vi "test_RxUDP.vi"() -> ()   [LabVIEW 2020]
uses:
  <instrlib>/AIM GmbH/_AIM 664/_controls/comm_computedMAC-IP.ctl
  <instrlib>/AIM GmbH/_AIM 664/_controls/comm_verification_rx.ctl
  <instrlib>/AIM GmbH/_AIM 664/_controls/comm_udp_rx.ctl
  <instrlib>/AIM GmbH/_AIM 664/bsp/Controls/IrigTime.ctl
  <instrlib>/AIM GmbH/_AIM 664/bsp/Fdx Create Session (Rx-VL-Oriented).vi
  <instrlib>/AIM GmbH/_AIM 664/bsp/Receive/FdxCreateRxVL.vi
  <instrlib>/AIM GmbH/_AIM 664/bsp/Fdx Create UDP Port (RX-CommPort).vi
  <instrlib>/AIM GmbH/_AIM 664/bsp/Fdx Start (Rx).vi
  <instrlib>/AIM GmbH/_AIM 664/bsp/TargetIndependentAdmin/FdxFwIrig2StructIrig.vi
  <instrlib>/AIM GmbH/_AIM 664/bsp/Fdx Stop (Rx).vi
  <instrlib>/AIM GmbH/_AIM 664/AIM664LV.lvlib
panel:
  out "IrigTime out":T1
  out "Udp Message":u8[](array[numeric]) format="%.0x"
  out "time stamp":timestamp
  out "timestamp s":dbl format="%#_15g"
  out "read time uS":u32(graph)
  out "MsgRead Total":u32=2
  in  "rx fetch rate mS":u32=100
  out "GlobalStat Out":T2={"TotalByteCount"=[139198, 0, 0, 0, 0, 0, 0, 0], "FrameGoodCount"=[1762, 0, 0, 0, 0, 0, 0, 0], "FrameErrorCount"=[0, 0, 0, 0, 0, 0, 0, 0], "BytesPerSecond"=[15800, 0, 0, 0, 0, 0, 0, 0], "FramesPerSecond"=[200, 0, 0, 0, 0, 0, 0, 0], "PhysErrorCount"=[0, 0, 0, 0, 0, 0, 0, 0], "PreamErrorCount"=[0, 0, 0, 0, 0, 0, 0, 0], "UnaligErrorCount"=[0, 0, 0, 0, 0, 0, 0, 0], "CRCErrorCount"=[0, 0, 0, 0, 0, 0, 0, 0], "IFGErrorCount"=[0, 0, 0, 0, 0, 0, 0, 0], "IPErrorCount"=[0, 0, 0, 0, 0, 0, 0, 0], "MACErrorCount"=[0, 0, 0, 0, 0, 0, 0, 0], "NoSfdErrorCount"=[0, 0, 0, 0, 0, 0, 0, 0], "VLLenErrorCount"=[0, 0, 0, 0, 0, 0, 0, 0], "SNIntegrityErrorCount"=[0, 0, 0, 0, 0, 0, 0, 0], "TrafShapingViolationCount"=[0, 0, 0, 0, 0, 0, 0, 0], "MAC1Short"=[0, 0, 0, 0, 0, 0, 0, 0], "MAC64To127Count"=[1762, 0, 0, 0, 0, 0, 0, 0], "MAC128To255Count"=[0, 0, 0, 0, 0, 0, 0, 0], "MAC256To511Count"=[0, 0, 0, 0, 0, 0, 0, 0], "MAC512To1023Count"=[0, 0, 0, 0, 0, 0, 0, 0], "MAC1024To1518Count"=[0, 0, 0, 0, 0, 0, 0, 0], "MACLong"=[0, 0, 0, 0, 0, 0, 0, 0]}
  in  "Control":u32(ring) items=["FDX_RX_GS_RES_NO_CNT", "FDX_RX_GS_RES_ALL_CNT", "FDX_RX_GS_RES_ERR_CNT"]
  out "MsgRead":u32=2
  out "MsgCount":u32=1762
  out "MsgErrorCount":u32
  out "RxStatus":u32=1
  out "Info":u32
  in  "stop":bool
  in  "Array":T3[](array[typedef])=[{"PortType"=enum."FDX_UDP_SAMPLING", "SubVIId"=1, "domainID"=1, "sideID"=1, "locationID"=1, "partitionID"=1, "UdpSrcPort"=24, "UdpDstPort"=23, "UdpNumBufMessages"=1, "UdpMaxMessageSize"=512, "UdpSamplingRate"=0}] {"partitionID" format="%.0b"}
  in  "VL Config":T4={"VlId"=60, "VLRange"=1, "VerificationMode"=0, "Bag"=0, "Jitter"=0, "MaxFrameLength"=0, "MaxSkew"=0, "VLBufSize"=32768, "FilterMode"=0, "FilterPosition"=0, "Padding"=0, "FilterMask"=0, "FilterData"=0, "MinFrameLength"=0} {"FilterMode" items=["FDX_RX_VL_FLT_DIS", "FDX_RX_VL_FLT_ENA ", "FDX_RX_VL_FLT_ENA_INV"]; "VLBufSize" format="%.0x"; "MaxFrameLength" format="%.0x"; "VerificationMode" items=["FDX_RX_VL_CHECK_ENA_DEFAULT"=65535, "FDX_RX_VL_CHECK_REDMAM"=16, "DX_RX_VL_CHECK_TRAFIC"=8, "FDX_RX_VL_CHECK_FRAMESIZE"=4, "FDX_RX_VL_CHECK_SNINTEG"=2, "FDX_RX_VL_CHECK_INVPAC"=1, "FDX_RX_VL_CHECK_DISA"=0]}
  out "computedAddresses":T5={"MACsrc"=[2, 0, 0, 1, 33, 32], "IPsrc"="10.1.33.1", "IPdest"="224.224.0.60"} {"MACsrc" format="%.0x"}
  in  "PortMap":u32=2
  out "PortInitOut":T6={"PortConfig"=0, "PortUsed"=1, "GlobalMemFree"=0, "SharedMemFree"=0} {"PortConfig" items=["FDX_SINGLE", "FDX_REDUNDANT"]}
  in  "port":u32
  in  "board":u32=1
  out "error out":errorcluster
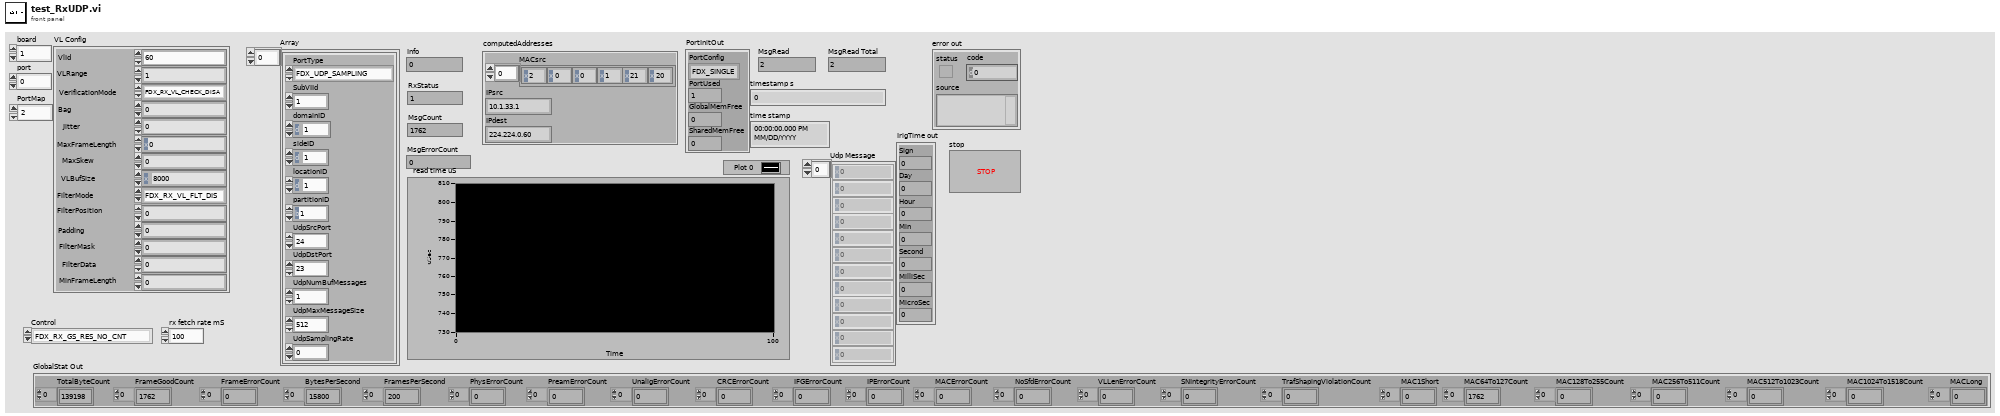
[diagram p1: front panel]
types:
  T1 = typedef "AIM664LV.lvlib/IrigTime.ctl" = cluster{"Sign":i32, "Day":u32, "Hour":u32, "Min":u32, "Second":u32, "MilliSec":u32, "MicroSec":u32}
  T2 = cluster{"TotalByteCount":u32[], "FrameGoodCount":u32[], "FrameErrorCount":u32[], "BytesPerSecond":u32[], "FramesPerSecond":u32[], "PhysErrorCount":u32[], "PreamErrorCount":u32[], "UnaligErrorCount":u32[], "CRCErrorCount":u32[], "IFGErrorCount":u32[], "IPErrorCount":u32[], "MACErrorCount":u32[], "NoSfdErrorCount":u32[], "VLLenErrorCount":u32[], "SNIntegrityErrorCount":u32[], "TrafShapingViolationCount":u32[], "MAC1Short":u32[], "MAC64To127Count":u32[], "MAC128To255Count":u32[], "MAC256To511Count":u32[], "MAC512To1023Count":u32[], "MAC1024To1518Count":u32[], "MACLong":u32[]}
  T3 = typedef "AIM664LV.lvlib/comm_udp_rx.ctl" = cluster{"PortType":enum16{"FDX_UDP_SAMPLING", "FDX_UDP_QUEUING"}, "SubVIId":u32, "domainID":u8, "sideID":u8, "locationID":u8, "partitionID":u8, "UdpSrcPort":u16, "UdpDstPort":u16, "UdpNumBufMessages":u32, "UdpMaxMessageSize":u32, "UdpSamplingRate":u32}
  T4 = typedef "AIM664LV.lvlib/comm_verification_rx.ctl" = cluster{"VlId":u16, "VLRange":u32, "VerificationMode":u32, "Bag":u32, "Jitter":u32, "MaxFrameLength":u32, "MaxSkew":u32, "VLBufSize":u32, "FilterMode":u32, "FilterPosition":u32, "Padding":u32, "FilterMask":u32, "FilterData":u32, "MinFrameLength":u32}
  T5 = typedef "AIM664LV.lvlib/comm_computedMAC-IP.ctl" = cluster{"MACsrc":u8[], "IPsrc":string, "IPdest":string}
  T6 = cluster{"PortConfig":u32, "PortUsed":u32, "GlobalMemFree":u32, "SharedMemFree":u32}
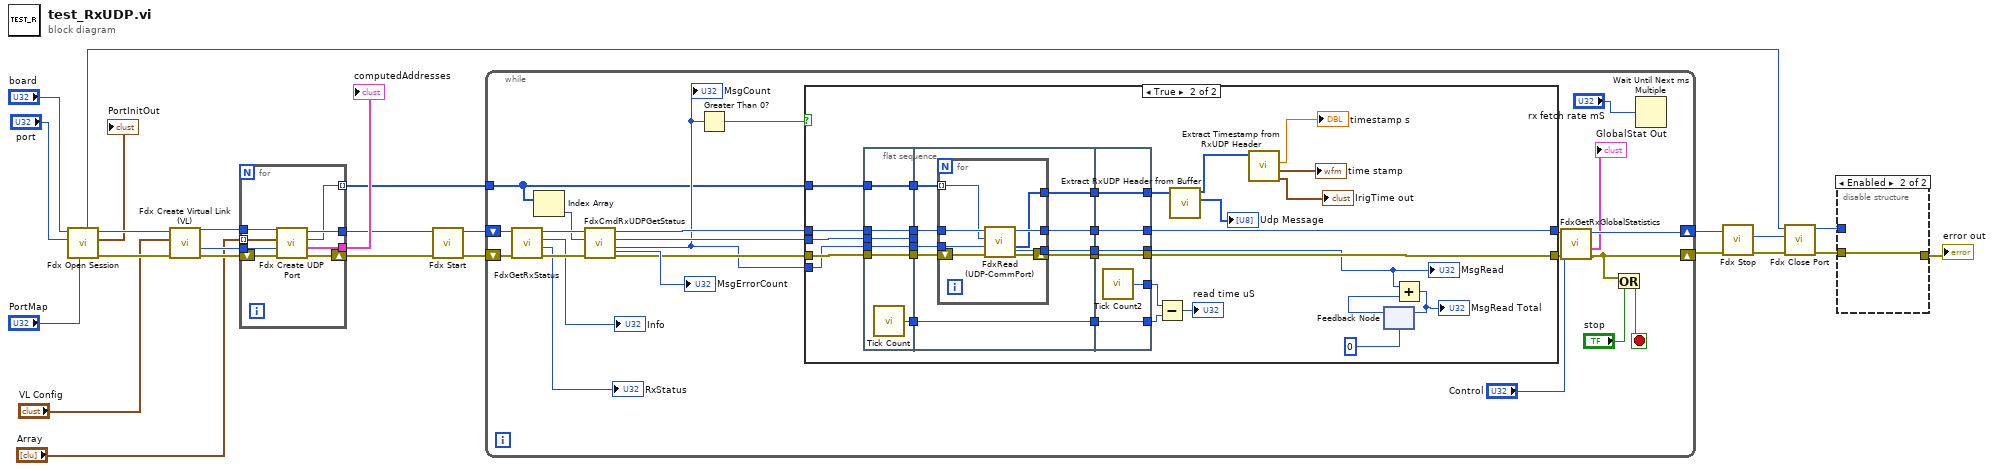
[diagram p0: block diagram]
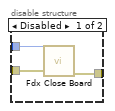
[diagram p2: hidden frame]
diagram:
  n1 = call-poly <instrlib>:"Fdx Open Session.vi"("PortMap"="PortMap", "port"="port", "board"="board") -> ("error out"=w25:errorcluster, "PortInitOut"=→"PortInitOut":T6, "InstrumentHandle_port out"=w20:u32, "InstrumentHandle_board out"=w19:u32)  [unwired: 3 in, 2 out]
  n2 = call-poly <instrlib>:"Fdx Create Virtual Link (VL).vi"("error in (no error)"=w25, "VL Config"="VL Config", "InstrumentHandle_port in"=w20) -> ("error out"=w24:errorcluster, "VlId"=w11:u16, "InstrumentHandle_port out"=w10:u32)  [unwired: 6 in]
  n3 = for {
    tunnel: w11 -> [w31]
    tunnel: w10 -> [w30]
    tunnel: [w29] -> w9
    tunnel: [w28] -> w7
    tunnel: [w27] -> w4 mode=indexing
    tunnel: "Array" -> [w26] mode=indexing
    shift-right: [w32] -> w23
    shift-left: w24 -> [w33]
    n4 = call-poly <instrlib>:"Fdx Create UDP Port.vi"("error in"=w33, "VlId"=w31, "CommPort Config"=w26, "port handle in"=w30) -> ("error out"=w32:errorcluster, "computedAddresses"=w29:T5, "commPort handle out"=w27:u32, "port handle out"=w28:u32)  [unwired: 4 in]
  }
  "computedAddresses" <- w9
  n5 = call-poly <instrlib>:"Fdx Start.vi"("error in"=w23, "InstrumentHandle_port in"=w7) -> ("error out"=w5:errorcluster, "InstrumentHandle_port out"=w6:u32)  [unwired: 8 in]
  n6 = while {
    shift-right: [w37] -> w3
    shift-left: w6 -> [w53]
    shift-right: [w38] -> w2
    shift-left: w5 -> [w52]
    tunnel: w4 -> [w34]
    stop <- w54 stop-if-true
    n7 = call <instrlib>:"FdxGetRxStatus.vi"("error in"=w52, "InstrumentHandle_port in"=w53) -> ("error out"=w51:errorcluster, "RxStatus"=→"RxStatus":u32, "Info"=→"Info":u32, "InstrumentHandle_port out"=w50:u32)  [unwired: 6 in]
    n8 = Index Array(array=w34) -> (element=w35:u32)  [unwired: 1 in]
    n9 = call <instrlib>:"FdxCmdRxUDPGetStatus.vi"("error in"=w51, "UdpHandle"=w35, "InstrumentHandle_port"=w50) -> ("error out"=w45:errorcluster, "MsgCount"=w42:u32, "UdpHandle Out"=w44:u32, "InstrumentHandle_port"=w43:u32, "MsgErrorCount"=→"MsgErrorCount":u32)  [unwired: 4 in]
    "MsgCount" <- w42
    n10 = Greater Than 0?(x=w42) -> (x > 0?=w46:bool)
    n11 = case shown="True" w46 {
      tunnel: w45 -> [w57 w87]
      tunnel: w44 -> [_ w89]
      tunnel: w43 -> [w58 w88]
      tunnel: [w58 w84] -> w40
      tunnel: [w57 w85] -> w41
      tunnel: w42 -> [_ w86]
      tunnel: w34 -> [_ w65]
      frame False {
      }
      frame True {
        n12 = flat-sequence {
          tunnel: w86 -> [w92]
          tunnel: w87 -> [w93]
          tunnel: w88 -> [w94]
          tunnel: w89 -> [w95]
          tunnel: [w95] -> w79
          tunnel: [w94] -> w78
          tunnel: [w93] -> w77
          tunnel: [w92] -> w76
          tunnel: [w91] -> w68
          tunnel: [w90] -> w66
          tunnel: w65 -> [w90]
          tunnel: w79 -> [_]
          tunnel: w78 -> [w104]
          tunnel: w77 -> [w103]
          tunnel: w76 -> [w102]
          tunnel: [w101] -> w75
          tunnel: [w100] -> w74
          tunnel: [w99] -> w73
          tunnel: [w98] -> w72
          tunnel: [w97] -> w69
          tunnel: w68 -> [w97]
          tunnel: w66 -> [w96]
          tunnel: [w115] -> w81
          tunnel: [w116] -> w64
          tunnel: [w117] -> w84
          tunnel: [w118] -> w85
          tunnel: w75 -> [w118]
          tunnel: w74 -> [w117]
          tunnel: w73 -> [w116]
          tunnel: w72 -> [w115]
          tunnel: [w114] -> w71
          tunnel: [w113] -> w70
          tunnel: w69 -> [w113]
          frame #0 {
            n13 = call "Tick Count"() -> ("Tick Count(uSec)"=w91:u32)
          }
          frame #1 {
            n14 = for {
              tunnel: w104 -> [w112]
              tunnel: w102 -> [w110]
              tunnel: [w108] -> w100
              tunnel: [w107] -> w99
              tunnel: [w106] -> w98
              shift-right: [w109] -> w101
              shift-left: w103 -> [w111]
              tunnel: w96 -> [w105] mode=indexing
              n15 = call <instrlib>:"FdxRead (UDP-CommPort).vi"("error in"=w111, "MsgCount"=w110, "UdpHandle"=w105, "InstrumentHandle_port"=w112) -> ("error out"=w109:errorcluster, "ReadBuffer"=w107:u8[], "InstrumentHandle_port"=w108:u32, "MsgRead"=w106:u32)  [unwired: 3 in, 1 out]
            }
          }
          frame #2 {
            n16 = call "Tick Count2"() -> ("Tick Count(uSec)"=w114:u32)
          }
        }
        n17 = Subtract(x=w71, y=w70) -> (x-y=→"read time uS":u32)
        n18 = call "Extract RxUDP Header from Buffer.vi"("ReadBuffer in"=w64) -> ("Udp Message"=→"Udp Message":u8[], "Header"=w63:u32[])  [unwired: 9 in]
        n19 = call "Extract Timestamp from RxUDP Header.vi"("header in"=w63) -> ("IrigTime out"=→"IrigTime out":T1, "time stamp out"=→"time stamp":timestamp, "seconds out"=→"timestamp s":dbl)  [unwired: 7 in, 1 out]
        n20 = feedback #1(u32 0 ("MsgRead")) -> (w82:u32)
        n21 = Add(x=w81, y=w82) -> (x+y=w80:u32)
        "MsgRead Total" <- w80
        n22 = feedback-in #1(w80) -> ()
        "MsgRead" <- w81
      }
    }
    n23 = call <instrlib>:"FdxGetRxGlobalStatistics.vi"("error in"=w41, "Control"="Control", "InstrumentHandle_port in"=w40) -> ("error out"=w38:errorcluster, "GlobalStat Out"=→"GlobalStat Out":T2, "InstrumentHandle_port out"=w37:u32)  [unwired: 6 in]
    n24 = Or(x=w38, y="stop") -> (x .or. y?=w54:bool)
    n25 = Wait Until Next ms Multiple(millisecond multiple="rx fetch rate mS") -> ()  [unwired: 1 out]
  }
  n26 = call-poly <instrlib>:"Fdx Stop.vi"("error in"=w2, "InstrumentHandle_port in"=w3) -> ("error out"=w22:errorcluster, "InstrumentHandle_port out"=w21:u32)  [unwired: 8 in]
  n27 = call <instrlib>:"Fdx Close Port.vi"("error in"=w22, "InstrumentHandle_port in"=w21, "InstrumentHandle_board in"=w19) -> ("error out"=w17:errorcluster, "InstrumentHandle_board out"=w16:u32)  [unwired: 7 in]
  n28 = disable-structure shown="Enabled" {
    disable-tunnel: w17 -> [w121 w122]
    disable-tunnel: w16 -> [w120 _]
    disable-tunnel: [w119 w122] -> w15
    frame Disabled {
      n29 = call <instrlib>:"Fdx Close Board.vi"("error in"=w121, "InstrumentHandle_board in"=w120) -> ("error out"=w119:errorcluster)  [unwired: 9 in]
    }
    frame Enabled {
    }
  }
  "error out" <- w15
